vi "TSCANfd_Table.vi"(6 "Message Name":string[][](array[string]), 7 "ms?":bool, 8 "SigValue":dbl[][](array[numeric]), 9 "SigName":string[][](array[string]), 10 "Messages":T1(array[cluster]), 11 "MCListbox reference handle":refnum<vi>) -> ()   [LabVIEW 2014]
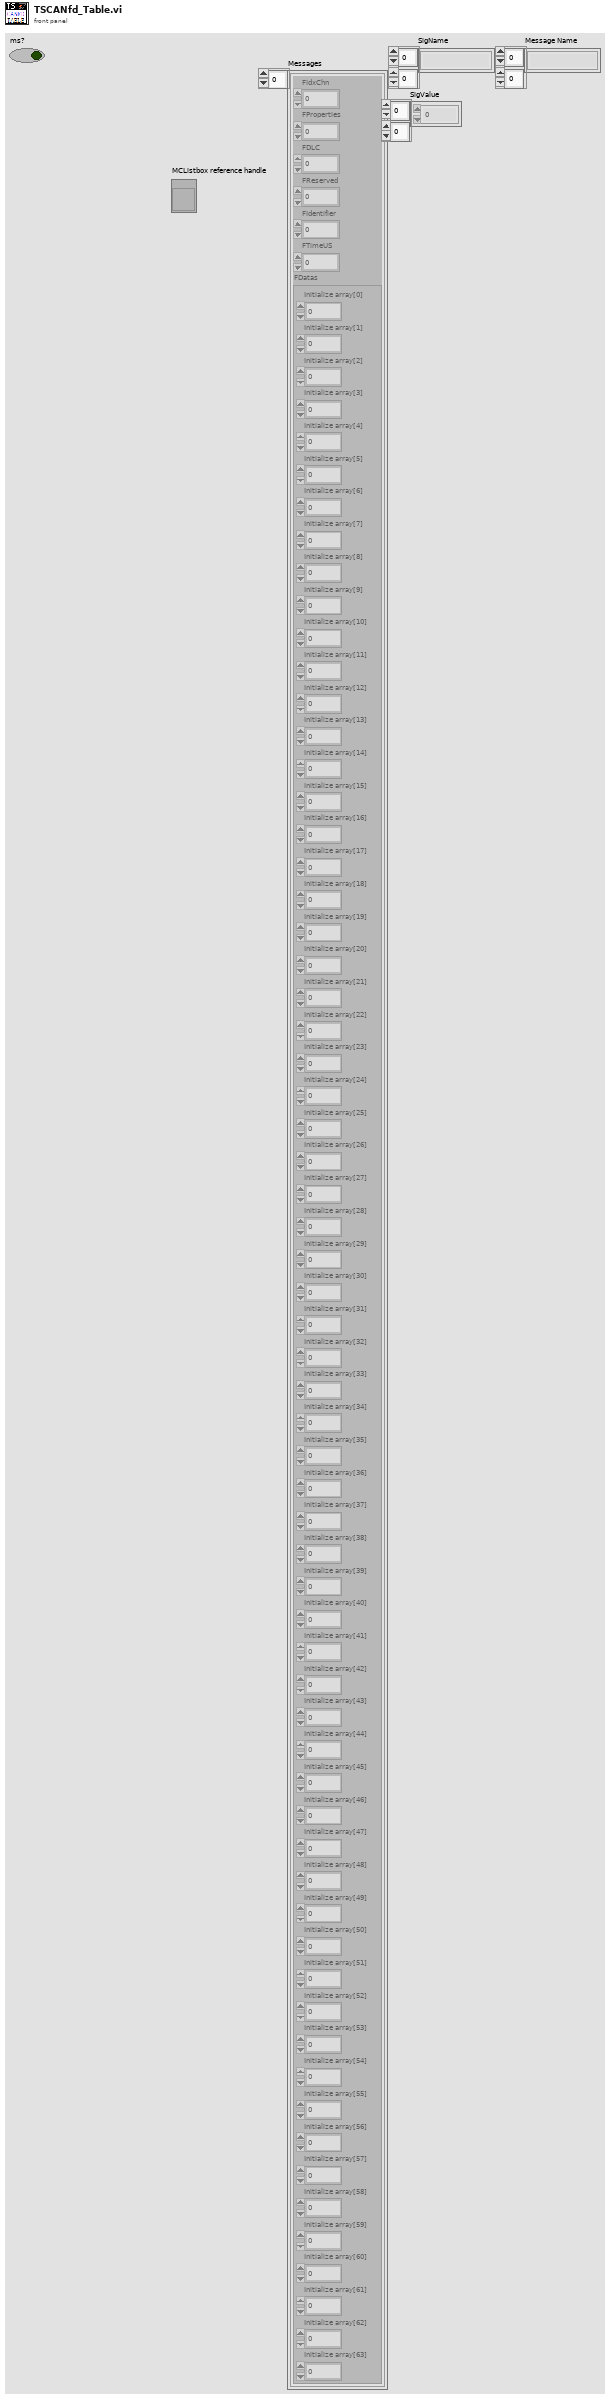
[diagram p1: front panel]
types:
  T1 = cluster{"FIdxChn":u8, "FProperties":u8, "FDLC":u8, "FReserved":u8, "FIdentifier":i32, "FTimeUS":u64, "FDatas":cluster{"Initialize array[0]":u8, "Initialize array[1]":u8, "Initialize array[2]":u8, "Initialize array[3]":u8, "Initialize array[4]":u8, "Initialize array[5]":u8, "Initialize array[6]":u8, "Initialize array[7]":u8, "Initialize array[8]":u8, "Initialize array[9]":u8, "Initialize array[10]":u8, "Initialize array[11]":u8, "Initialize array[12]":u8, "Initialize array[13]":u8, "Initialize array[14]":u8, "Initialize array[15]":u8, "Initialize array[16]":u8, "Initialize array[17]":u8, "Initialize array[18]":u8, "Initialize array[19]":u8, "Initialize array[20]":u8, "Initialize array[21]":u8, "Initialize array[22]":u8, "Initialize array[23]":u8, "Initialize array[24]":u8, "Initialize array[25]":u8, "Initialize array[26]":u8, "Initialize array[27]":u8, "Initialize array[28]":u8, "Initialize array[29]":u8, "Initialize array[30]":u8, "Initialize array[31]":u8, "Initialize array[32]":u8, "Initialize array[33]":u8, "Initialize array[34]":u8, "Initialize array[35]":u8, "Initialize array[36]":u8, "Initialize array[37]":u8, "Initialize array[38]":u8, "Initialize array[39]":u8, "Initialize array[40]":u8, "Initialize array[41]":u8, "Initialize array[42]":u8, "Initialize array[43]":u8, "Initialize array[44]":u8, "Initialize array[45]":u8, "Initialize array[46]":u8, "Initialize array[47]":u8, "Initialize array[48]":u8, "Initialize array[49]":u8, "Initialize array[50]":u8, "Initialize array[51]":u8, "Initialize array[52]":u8, "Initialize array[53]":u8, "Initialize array[54]":u8, "Initialize array[55]":u8, "Initialize array[56]":u8, "Initialize array[57]":u8, "Initialize array[58]":u8, "Initialize array[59]":u8, "Initialize array[60]":u8, "Initialize array[61]":u8, "Initialize array[62]":u8, "Initialize array[63]":u8}}[]
  T2 = cluster{"Initialize array[0]":u8, "Initialize array[1]":u8, "Initialize array[2]":u8, "Initialize array[3]":u8, "Initialize array[4]":u8, "Initialize array[5]":u8, "Initialize array[6]":u8, "Initialize array[7]":u8, "Initialize array[8]":u8, "Initialize array[9]":u8, "Initialize array[10]":u8, "Initialize array[11]":u8, "Initialize array[12]":u8, "Initialize array[13]":u8, "Initialize array[14]":u8, "Initialize array[15]":u8, "Initialize array[16]":u8, "Initialize array[17]":u8, "Initialize array[18]":u8, "Initialize array[19]":u8, "Initialize array[20]":u8, "Initialize array[21]":u8, "Initialize array[22]":u8, "Initialize array[23]":u8, "Initialize array[24]":u8, "Initialize array[25]":u8, "Initialize array[26]":u8, "Initialize array[27]":u8, "Initialize array[28]":u8, "Initialize array[29]":u8, "Initialize array[30]":u8, "Initialize array[31]":u8, "Initialize array[32]":u8, "Initialize array[33]":u8, "Initialize array[34]":u8, "Initialize array[35]":u8, "Initialize array[36]":u8, "Initialize array[37]":u8, "Initialize array[38]":u8, "Initialize array[39]":u8, "Initialize array[40]":u8, "Initialize array[41]":u8, "Initialize array[42]":u8, "Initialize array[43]":u8, "Initialize array[44]":u8, "Initialize array[45]":u8, "Initialize array[46]":u8, "Initialize array[47]":u8, "Initialize array[48]":u8, "Initialize array[49]":u8, "Initialize array[50]":u8, "Initialize array[51]":u8, "Initialize array[52]":u8, "Initialize array[53]":u8, "Initialize array[54]":u8, "Initialize array[55]":u8, "Initialize array[56]":u8, "Initialize array[57]":u8, "Initialize array[58]":u8, "Initialize array[59]":u8, "Initialize array[60]":u8, "Initialize array[61]":u8, "Initialize array[62]":u8, "Initialize array[63]":u8}
  T3 = typedef "LVRowAndColumnUnsignedTypeDef.ctl" = cluster{"Row":u32, "Column":u32}
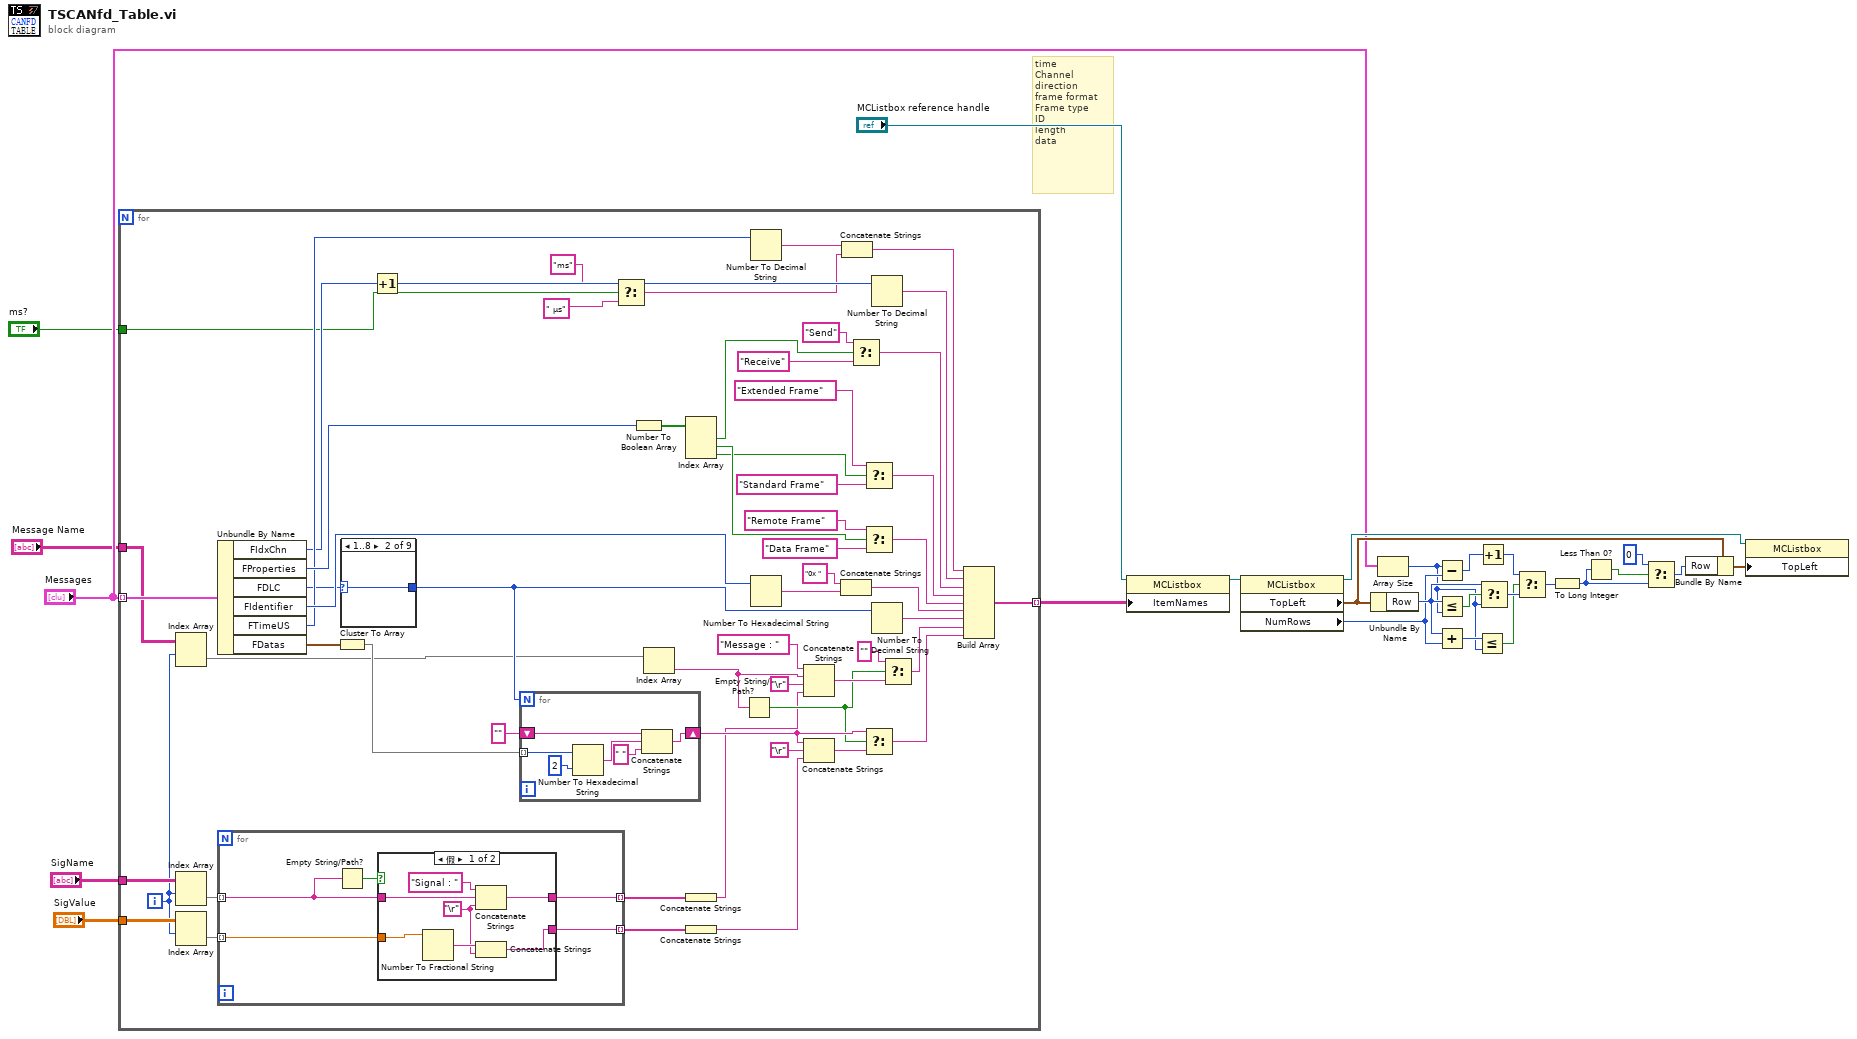
[diagram p0: block diagram]
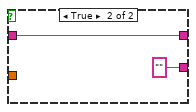
[diagram p2: hidden frame]
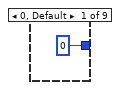
[diagram p3: hidden frame]
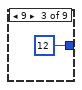
[diagram p4: hidden frame]
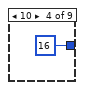
[diagram p5: hidden frame]
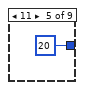
[diagram p6: hidden frame]
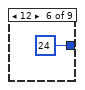
[diagram p7: hidden frame]
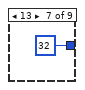
[diagram p8: hidden frame]
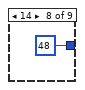
[diagram p9: hidden frame]
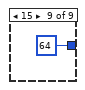
[diagram p10: hidden frame]
diagram:
  # "time\nChannel\ndirection\nframe format\nFrame type\nID\nlength\ndata"
  n1 = for {
    tunnel: "Messages" -> [w83] mode=indexing
    tunnel: [w60] -> w25 mode=indexing
    tunnel: "SigName" -> [w50]
    tunnel: "SigValue" -> [w37]
    tunnel: "Message Name" -> [w49]
    tunnel: "ms?" -> [w29]
    i -> [w30]
    n2 = Index Array(array=w49, index (row)=w30) -> (element=w33:string[])  [unwired: 1 in]
    n3 = Index Array(array=w50, index (row)=w30) -> (element=w32:string[])  [unwired: 1 in]
    n4 = Index Array(array=w37, index (row)=w30) -> (element=w31:dbl[])  [unwired: 1 in]
    n5 = Unbundle By Name(w83) -> ("FIdxChn"=w59:u8, "FProperties"=w82:u8, "FDLC"=w52:u8, "FIdentifier"=w71:i32, "FTimeUS"=w70:u64, "FDatas"=w68:T2)
    n6 = for {
      tunnel: w32 -> [w88] mode=indexing
      tunnel: [w87] -> w44 mode=indexing
      tunnel: w31 -> [w85] mode=indexing
      tunnel: [w84] -> w36 mode=indexing
      n7 = Empty String/Path?(string/path=w88) -> (empty?=w86:bool)
      n8 = case shown="假" w86 {
        tunnel: w88 -> [w95 w97]
        tunnel: [w94 w97] -> w87
        tunnel: w85 -> [w92 _]
        tunnel: [w89 ""] -> w84
        frame False {
          w90 = "\r"
          n9 = Number To Fractional String(number=w92) -> (F-format string=w91:string)  [unwired: 3 in]
          n10 = Concatenate Strings("Signal : " ("字符串"), w95, w90) -> (w94:string)
          n11 = Concatenate Strings(w91, w90) -> (w89:string)
        }
        frame True {
        }
      }
    }
    n12 = Cluster To Array(cluster=w68) -> (array=w67:u8[])
    n13 = case shown="1..8" w52 {
      selector: w52 -> [_ w99 _ _ _ _ _ _ _]
      tunnel: [0 ("CANFD DLC") w99 12 ("CANFD DLC") 16 ("CANFD DLC") 20 ("CANFD DLC") 24 ("CANFD DLC") 32 ("CANFD DLC") 48 ("CANFD DLC") 64 ("CANFD DLC")] -> w51
      frame 0, Default {
      }
      frame 1..8 {
      }
      frame 9 {
      }
      frame 10 {
      }
      frame 11 {
      }
      frame 12 {
      }
      frame 13 {
      }
      frame 14 {
      }
      frame 15 {
      }
    }
    n14 = Increment(x=w59) -> (x+1=w58:u8)
    n15 = for {
      N: w51 -> [_]
      tunnel: w67 -> [w109] mode=indexing
      shift-right: [w111] -> w61
      shift-left: "" -> [w112]
      n16 = Number To Hexadecimal String(1:i16 2 ("width (-)"), 2:w109) -> (0:w108:string)
      n17 = Concatenate Strings(w112, w108, " " ("string")) -> (w111:string)
    }
    n18 = Select(t="ms" ("字符串"), s=w29, f=" μs" ("字符串")) -> (s? t:f=w26:string)
    n19 = Number To Boolean Array(number=w82) -> (Boolean array=w81:bool[])
    n20 = Index Array(array=w33) -> (element=w46:string)  [unwired: 1 in]
    n21 = Index Array(array=w81) -> (element #1=w80:bool, element #2=w75:bool, element #3=w72:bool)  [unwired: 3 in]
    n22 = Concatenate Strings(w44) -> (w35:string)
    n23 = Concatenate Strings(w36) -> (w34:string)
    n24 = Empty String/Path?(string/path=w46) -> (empty?=w41:bool)
    n25 = Number To Decimal String(number=w70) -> (decimal integer string=w53:string)  [unwired: 1 in]
    n26 = Number To Hexadecimal String(2:w71) -> (0:w56:string)  [unwired: 1 in]
    n27 = Concatenate Strings("Message : " ("字符串"), w46, "\r", w35) -> (w43:string)
    n28 = Concatenate Strings(w61, "\r", w34) -> (w40:string)
    n29 = Concatenate Strings("0x " ("字符串"), w56) -> (w57:string)
    n30 = Concatenate Strings(w53, w26) -> (w54:string)
    n31 = Select(t="Send", s=w80, f="Receive") -> (s? t:f=w65:string)
    n32 = Select(t="Extended Frame", s=w72, f="Standard Frame") -> (s? t:f=w64:string)
    n33 = Select(t="Remote Frame", s=w75, f="Data Frame") -> (s? t:f=w63:string)
    n34 = Select(t=w61, s=w41, f=w40) -> (s? t:f=w39:string)
    n35 = Number To Decimal String(number=w58) -> (decimal integer string=w66:string)  [unwired: 1 in]
    n36 = Number To Decimal String(number=w51) -> (decimal integer string=w62:string)  [unwired: 1 in]
    n37 = Select(t="", s=w41, f=w43) -> (s? t:f=w48:string)
    n38 = Build Array(w54, w66, w65, w64, w63, w57, w62, w48, w39) -> (w60:string[])
  }
  n39 = property class="MCListbox"(reference="MCListbox reference handle", "ItemNames"=w25) -> (reference out=w6:refnum<vi>)  [unwired: 1 in, 1 out]
  n40 = property class="MCListbox"(reference=w6) -> (reference out=w14:refnum<vi>, "TopLeft"=w13:T3, "NumRows"=w21:u32)  [unwired: 1 in, 1 out]
  n41 = Unbundle By Name(w13) -> ("Row"=w22:u32)
  n42 = Array Size(array="Messages") -> (size(s)=w19:i32)
  n43 = Subtract(x=w19, y=w21) -> (x-y=w18:u32)
  n44 = Less Or Equal?(x=w22, y=w19) -> (x <= y?=w23:bool)
  n45 = Add(x=w22, y=w21) -> (x+y=w20:u32)
  n46 = Less Or Equal?(x=w20, y=w19) -> (x <= y?=w15:bool)
  n47 = Increment(x=w18) -> (x+1=w16:u32)
  n48 = Select(t=w22, s=w23, f=w19) -> (s? t:f=w17:u32)
  n49 = Select(t=w16, s=w15, f=w17) -> (s? t:f=w12:u32)
  n50 = To Long Integer(number=w12) -> (32bit integer=w10:i32)
  n51 = Less Than 0?(x=w10) -> (x < 0?=w11:bool)
  n52 = Select(t=0, s=w11, f=w10) -> (s? t:f=w9:i32)
  n53 = Bundle By Name(cluster=w13, "Row"=w9) -> (w7:T3)
  n54 = property class="MCListbox"(reference=w14, "TopLeft"=w7) -> ()  [unwired: 1 in, 2 out]
